vi "foot_on_line.vi"(1 "dot":cluster{"X":sgl, "Y":sgl}={"X"=100.0, "Y"=100.0}, 2 "line end":cluster{"X":sgl, "Y":sgl}={"X"=100.0, "Y"=100.0}, 3 "line start":cluster{"X":sgl, "Y":sgl}={"X"=100.0, "Y"=100.0}) -> (0 "foot on line？":bool)   [LabVIEW 2018]
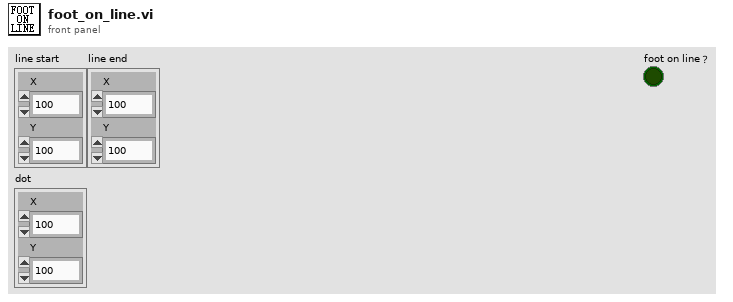
[diagram p1: front panel]
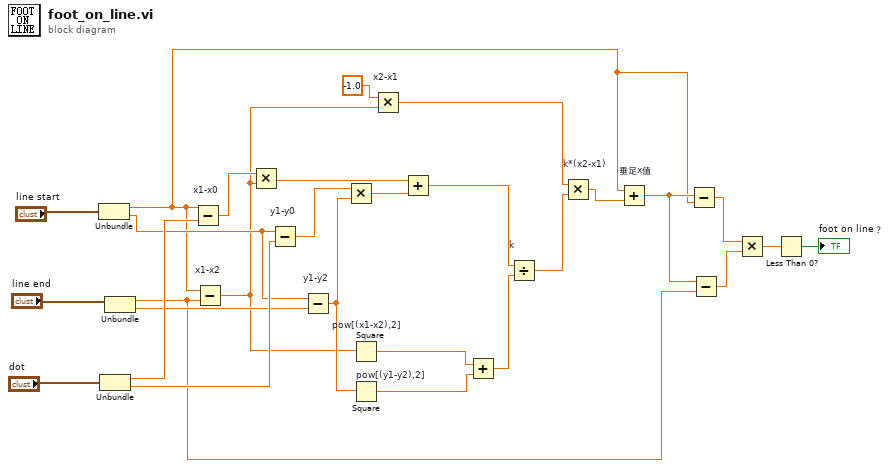
[diagram p0: block diagram]
diagram:
  n1 = Unbundle("line start") -> ("X"=w6:sgl, "Y"=w23:sgl)
  n2 = Unbundle("dot") -> ("X"=w25:sgl, "Y"=w24:sgl)
  n3 = Unbundle("line end") -> ("X"=w5:sgl, "Y"=w22:sgl)
  n4 = Subtract "x1-x0"(x=w6, y=w25) -> (x-y=w21:sgl)
  n5 = Subtract "x1-x2"(x=w6, y=w5) -> (x-y=w11:sgl)
  n6 = Multiply(x=w21, y=w11) -> (x*y=w18:sgl)
  n7 = Subtract "y1-y0"(x=w23, y=w24) -> (x-y=w20:sgl)
  n8 = Subtract "y1-y2"(x=w23, y=w22) -> (x-y=w17:sgl)
  n9 = Multiply(x=w20, y=w17) -> (x*y=w19:sgl)
  n10 = Square "pow[(x1-x2),2]"(x=w11) -> (x^2=w16:sgl)
  n11 = Square "pow[(y1-y2),2]"(x=w17) -> (x^2=w15:sgl)
  n12 = Multiply "x2-x1"(x=-1.0 ("y"), y=w11) -> (x*y=w10:dbl)
  n13 = Add(x=w18, y=w19) -> (x+y=w14:sgl)
  n14 = Add(x=w16, y=w15) -> (x+y=w13:sgl)
  n15 = Divide "k"(x=w14, y=w13) -> (x/y=w9:sgl)
  n16 = Multiply "k*(x2-x1)"(x=w10, y=w9) -> (x*y=w8:dbl)
  n17 = Add "垂足x值"(x=w6, y=w8) -> (x+y=w7:dbl)
  n18 = Subtract(x=w7, y=w6) -> (x-y=w4:dbl)
  n19 = Subtract(x=w7, y=w5) -> (x-y=w3:dbl)
  n20 = Multiply(x=w4, y=w3) -> (x*y=w2:dbl)
  n21 = Less Than 0?(x=w2) -> (x < 0?=→"foot on line？":bool)
